vi "Default Section.vi"(8 "error in (no error)":errorcluster, 11 "Node Ptr":T1 format="%.0x") -> (0 "error out":errorcluster)   [LabVIEW 2019, in "Diagnostics Addon System Explorer.lvlib"]
uses:
  Diagnostics Addon System Explorer.lvlib
  <vilib>/NI VeriStand/Custom Device API/Custom Device Item Ref.ctl
  Addon Shared/SubVIs/Constants.vi
  <vilib>/NI VeriStand/Custom Device Tools/Custom Device Utility Library/NI VeriStand - Search for Item by GUID.vi
  <vilib>/NI VeriStand/Custom Device API/Custom Device API.lvlib
  <vilib>/NI VeriStand/Custom Device Tools/Custom Device Utility Library/Custom Device Utility Library.lvlib
  Addon Shared/Diagnostics Addon Shared.lvlib
panel:
  in  "SHDocVw.IWebBrowser":refnum<k7>(container)
  in  "Settings 6":i64 format="%.0x"
  in  "Settings 5":i64 format="%.0x"
  in  "Settings 4":i64 format="%.0x"
  in  "Settings 3":i64 format="%.0x"
  in  "Settings 2":i64 format="%.0x"
  in  "Settings 1":i64 format="%.0x"
  in  "Header 2":cluster{"Section Name":string}={"Section Name"="Section Default Values"}
  in  "Header":cluster{"Section Name":string}={"Section Name"="Section Item Settings"}
  in  "Description":string
  out "Name":string
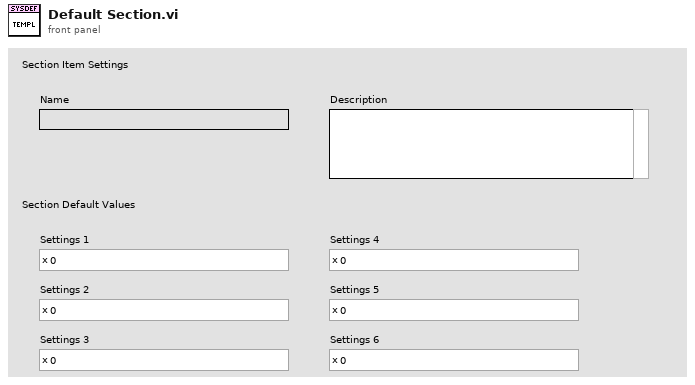
[diagram p1: front panel]
types:
  T1 = typedef "Custom Device API.lvlib/Custom Device Item Ref.ctl" = u64
  T2 = typedef "Custom Device API.lvlib/Custom Device Item Info.ctl" = cluster{"Name":string, "Is Channel":bool, "GUID":string, "Is Waveform":bool}
  T3 = typedef "Custom Device API.lvlib/Custom Device Channel.ctl" = cluster{"Type":T4, "Units":string, "Default Value":dbl, "Faultable":bool, "Scalable":bool}
  T4 = typedef "Custom Device API.lvlib/Custom Device Channel Type.ctl" = enum16{"Input", "Output"}
  T5 = typedef "Custom Device API.lvlib/Custom Device Commands.ctl" = enum16{"Default", "Item renamed", "Shutdown", "Dynamic button pressed"}
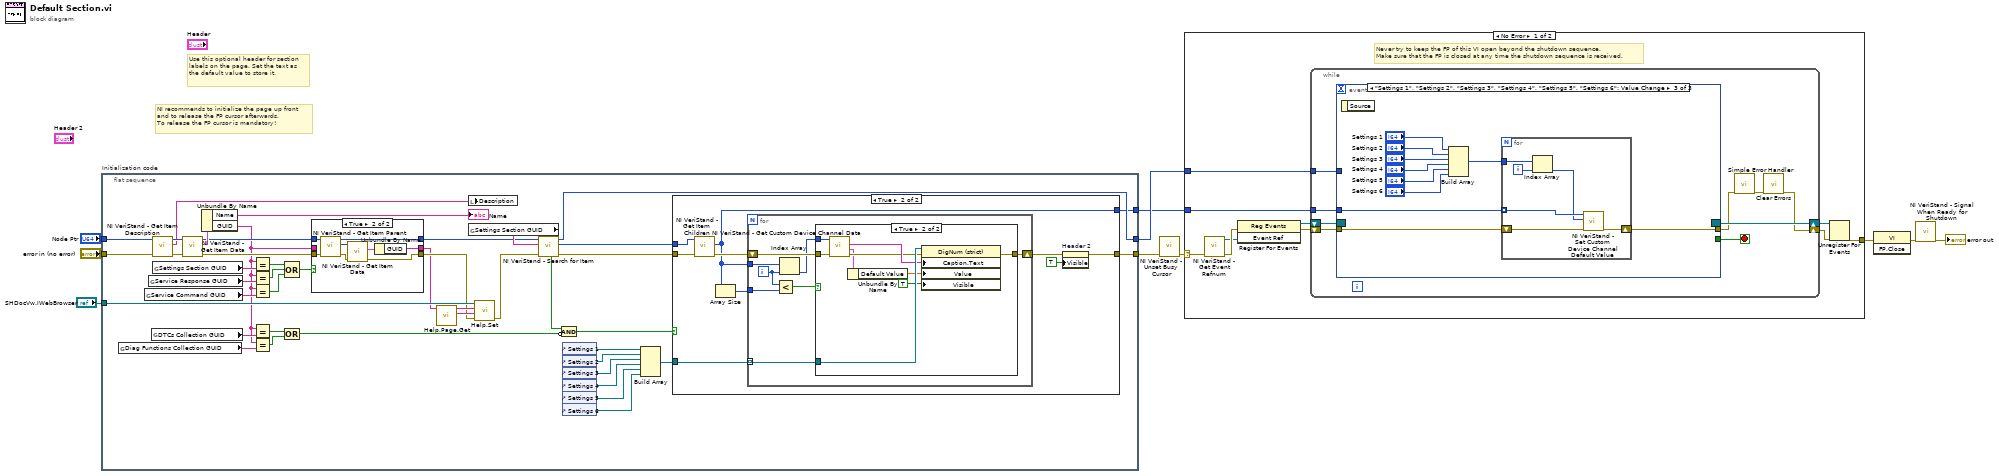
[diagram p0: block diagram]
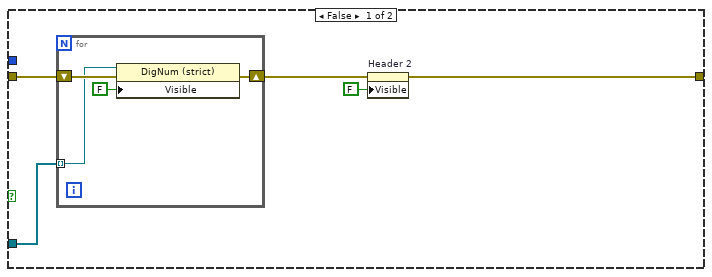
[diagram p3: hidden frame]
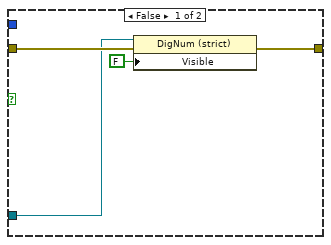
[diagram p4: hidden frame]
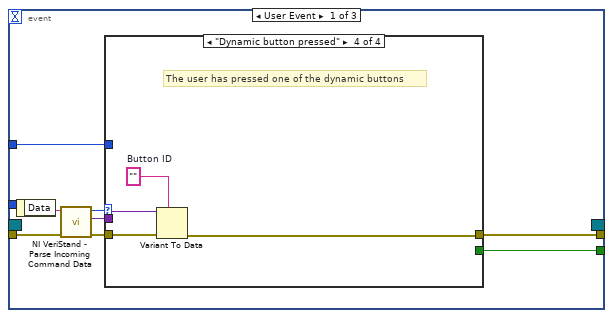
[diagram p5: hidden frame]
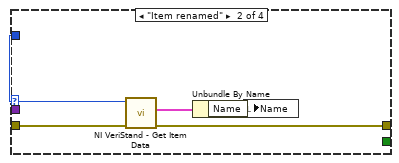
[diagram p7: hidden frame]
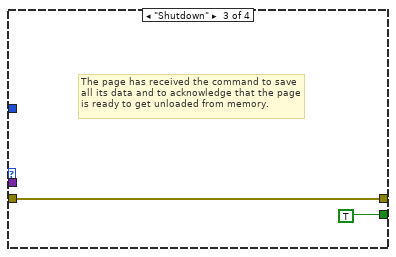
[diagram p8: hidden frame]
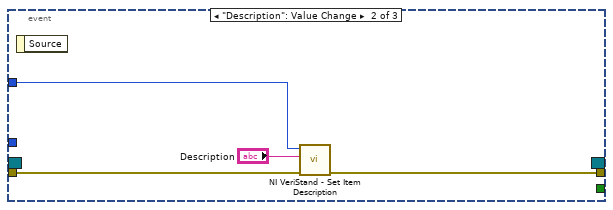
[diagram p9: hidden frame]
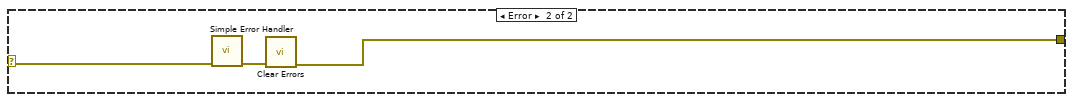
[diagram p10: hidden frame]
diagram:
  # "Use this optional header for section labels on the page. Set the text as the default value to store it."
  # "NI recommends to initialize the page up front\nand to release the FP cursor afterwards.\nTo release the FP cursor is mandatory!"
  n1 = flat-sequence "Initialization code" {
    tunnel: "error in (no error)" -> [w53]
    tunnel: "Node Ptr" -> [w52]
    tunnel: [w38] -> w6
    tunnel: [w37] -> w3
    tunnel: [w35] -> w2
    tunnel: "SHDocVw.IWebBrowser" -> [w33]
    frame #0 {
      n2 = global read "Constants.vi" "Diag Functions Collection GUID"() -> (w15:string)
      n3 = global read "Constants.vi" "Service Command GUID"() -> (w24:string)
      n4 = global read "Constants.vi" "Service Response GUID"() -> (w25:string)
      n5 = global read "Constants.vi" "DTCs Collection GUID"() -> (w16:string)
      n6 = call <vilib>:"NI VeriStand - Get Item Description.vi"("error in (no error)"=w53, "Item Ref in"=w52) -> ("error out"=w50:errorcluster, "Description"=w51:string, "Item Ref out"=w54:T1)  [unwired: 7 out]
      n7 = global read "Constants.vi" "Settings Section GUID"() -> (w23:string)
      n8 = call <vilib>:"NI VeriStand - Get Item Data.vi"("error in (no error)"=w50, "Item Ref in"=w54) -> ("error out"=w30:errorcluster, "Item Info"=w49:T2, "Item Ref out"=w29:T1)  [unwired: 7 out]
      n9 = Unbundle By Name(w49) -> ("Name"=→"Name":string, "GUID"=w14:string)
      n10 = Equal?(x=w14, y=w23) -> (x = y?=w20:bool)
      n11 = Equal?(x=w14, y=w25) -> (x = y?=w22:bool)
      n12 = Equal?(x=w14, y=w24) -> (x = y?=w21:bool)
      n13 = Equal?(x=w14, y=w16) -> (x = y?=w18:bool)
      n14 = Equal?(x=w14, y=w15) -> (x = y?=w17:bool)
      n15 = Compound Arithmetic op=OR(w20, w22, w21) -> (w19:bool)
      n16 = Compound Arithmetic op=OR(w18, w17) -> (w13:bool)
      n17 = case shown="True" w19 {
        tunnel: w30 -> [w57 w65]
        tunnel: w29 -> [w56 w64]
        tunnel: [w56 w63] -> w28
        tunnel: [w57 w59] -> w27
        tunnel: [w55 w58] -> w26
        tunnel: w14 -> [w55 _]
        frame False {
        }
        frame True {
          n18 = call <vilib>:"NI VeriStand - Get Item Parent.vi"("error in (no error)"=w65, "Item Ref in"=w64) -> ("error out"=w61:errorcluster, "Parent Ref"=w62:T1, "Item Ref out"=w63:T1)  [unwired: 6 in, 1 out]
          n19 = call <vilib>:"NI VeriStand - Get Item Data.vi"("error in (no error)"=w61, "Item Ref in"=w62) -> ("error out"=w59:errorcluster, "Item Info"=w60:T2)  [unwired: 8 out]
          n20 = Unbundle By Name(w60) -> ("GUID"=w58:string)
        }
      }
      n21 = call "Help.Page.Get.vi"("GUID"=w26) -> ("HTML File"=w34:string, "Main CHM File"=w31:string)  [unwired: 9 in]
      n22 = local write "Description"(w51) -> ()
      n23 = global read "Constants.vi" "Settings Section GUID"() -> (w47:string)
      n24 = call "Help.Set.vi"("error in (no error)"=w27, "HTML File"=w34, "Main CHM File"=w31, "SHDocVw.IWebBrowser2"=w33) -> ("error out"=w32:errorcluster)  [unwired: 7 in]
      n25 = call-poly <vilib>:"NI VeriStand - Search for Item.vi"("error in"=w32, "Item GUID"=w47, "Section Ref in"=w28) -> ("error out"=w39:errorcluster, "Item Ref"=w36:T1, "Section Ref out"=w37:T1, "Found"=w12:bool)  [unwired: 5 in]
      n26 = Compound Arithmetic op=AND(w12, invert w13) -> (w11:bool)
      n27 = control-ref of="Settings 1"() -> (w46:refnum<vi>)
      n28 = control-ref of="Settings 2"() -> (w45:refnum<vi>)
      n29 = control-ref of="Settings 3"() -> (w44:refnum<vi>)
      n30 = control-ref of="Settings 4"() -> (w43:refnum<vi>)
      n31 = control-ref of="Settings 5"() -> (w42:refnum<vi>)
      n32 = control-ref of="Settings 6"() -> (w41:refnum<vi>)
      n33 = Build Array(w46, w45, w44, w43, w42, w41) -> (w40:refnum<vi>[])
      n34 = case shown="True" w11 {
        tunnel: w40 -> [w70 w83]
        tunnel: w39 -> [w69 w82]
        tunnel: [w66 w75] -> w38
        tunnel: w36 -> [_ w80]
        tunnel: [_ w78] -> w35
        frame False {
          n35 = for {
            tunnel: w70 -> [w73] mode=indexing
            shift-right: [w71] -> w67
            shift-left: w69 -> [w74]
            n36 = property class="DigNum (strict)"(reference=w73, error in=w74, "Visible"=FALSE) -> (error out=w71:errorcluster)  [unwired: 1 out]
          }
          n37 = property on="Header 2" class="Clust (strict)"(error in=w67, "Visible"=FALSE) -> (error out=w66:errorcluster)  [unwired: 1 in, 1 out]
        }
        frame True {
          n38 = call <vilib>:"NI VeriStand - Get Item Children.vi"("error in (no error)"=w82, "Item Ref in"=w80) -> ("error out"=w81:errorcluster, "Child Refs"=w78:T1[])  [unwired: 6 in, 2 out]
          n39 = Array Size(array=w78) -> (size(s)=w79:i32)
          n40 = for {
            tunnel: w83 -> [w91] mode=indexing
            shift-right: [w90] -> w76
            shift-left: w81 -> [w88]
            tunnel: w78 -> [w89]
            tunnel: w79 -> [w85]
            i -> [w86]
            n41 = Less?(x=w86, y=w85) -> (x < y?=w84:bool)
            n42 = Index Array(array=w89, index=w86) -> (element=w87:T1)
            n43 = case shown="True" w84 {
              tunnel: w91 -> [w92 w104]
              tunnel: [w93 w103] -> w90
              tunnel: w88 -> [w94 w101]
              tunnel: w87 -> [_ w100]
              frame False {
                n44 = property class="DigNum (strict)"(reference=w92, error in=w94, "Visible"=FALSE) -> (error out=w93:errorcluster)  [unwired: 1 out]
              }
              frame True {
                n45 = call <vilib>:"NI VeriStand - Get Custom Device Channel Data.vi"("error in (no error)"=w101, "Channel Ref in"=w100) -> ("error out"=w98:errorcluster, "Channel"=w97:T3, "Channel Name"=w99:string)  [unwired: 4 in, 3 out]
                n46 = Unbundle By Name(w97) -> ("Default Value"=w96:dbl)
                n47 = property class="DigNum (strict)"(reference=w104, error in=w98, "Caption.Text"=w99, "Value"=w96, "Visible"=TRUE) -> (error out=w103:errorcluster)  [unwired: 1 out]
              }
            }
          }
          n48 = property on="Header 2" class="Clust (strict)"(error in=w76, "Visible"=TRUE) -> (error out=w75:errorcluster)  [unwired: 1 in, 1 out]
        }
      }
    }
  }
  n49 = call <vilib>:"NI VeriStand - Unset Busy Cursor.vi"("error in (no error)"=w6) -> ("error out"=w5:errorcluster)  [unwired: 10 out]
  n50 = case shown="No Error" w5 {
    selector: w5 -> [w106 w166]
    tunnel: [w111 w164] -> w10
    tunnel: w3 -> [w107 _]
    tunnel: w2 -> [w105 _]
    frame No Error {
      # "Never try to keep the FP of this VI open beyond the shutdown sequence.\nMake sure that the FP is closed at any time the shutdown sequence is received."
      n51 = call <vilib>:"NI VeriStand - Get Event Refnum.vi"("error in (no error)"=w106) -> ("error out"=w114:errorcluster, "Event Ref"=w110:refnum<user-event>)  [unwired: 9 out]
      n52 = register-events(error in=w114, w110) -> (reference out=w108:refnum<event-registration>, error out=w109:errorcluster)  [unwired: 1 in]
      n53 = while {
        tunnel: w107 -> [w119]
        shift-right: [w116] -> w112
        shift-left: w109 -> [w122]
        shift-right: [w123] -> w113
        shift-left: w108 -> [w121]
        tunnel: w105 -> [w115]
        stop <- w120 stop-if-true
        n54 = event shown="[2] \"Settings 1\", \"Settings 2\", \"Settings 3\", \"Settings 4\", \"Settings 5\", \"Settings 6\": Value Change" {
          selector: w121 -> [_ _ _]
          dyn-events: [_ _ _] -> w123
          timeout: _ -> [_ _ _]
          tunnel: w122 -> [w131 w146 w157]
          tunnel: [w127 _ _] -> w120
          tunnel: [w126 w145 w155] -> w118
          tunnel: w119 -> [w125 w147 _]
          tunnel: w115 -> [_ _ w156]
          event User Event {
            n55 = event-data() -> ("Data"=w130:string)  [unwired: 1 out]
            n56 = call <vilib>:"NI VeriStand - Parse Incoming Command Data.vi"("error in (no error)"=w131, "Incoming data"=w130) -> ("error out"=w129:errorcluster, "Outgoing data"=w124:variant, "Action"=w128:T5)  [unwired: 7 out]
            n57 = case shown="\"Dynamic button pressed\"" w128 {
              tunnel: w129 -> [w132 w137 w138 w143]
              tunnel: [_ _ TRUE _] -> w127
              tunnel: [w132 w134 w138 w140] -> w126
              tunnel: w125 -> [_ w136 _ _]
              tunnel: w124 -> [_ _ _ w142]
              frame "Default", Default {
              }
              frame "Item renamed" {
                n58 = call <vilib>:"NI VeriStand - Get Item Data.vi"("error in (no error)"=w137, "Item Ref in"=w136) -> ("error out"=w134:errorcluster, "Item Info"=w135:T2)  [unwired: 8 out]
                n59 = Unbundle By Name(w135) -> ("Name"=w133:string)
                n60 = local write "Name"(w133) -> ()
              }
              frame "Shutdown" {
                # "The page has received the command to save all its data and to acknowledge that the page is ready to get unloaded from memory."
              }
              frame "Dynamic button pressed" {
                w141 = ""  # Button ID
                # "The user has pressed one of the dynamic buttons"
                n61 = Variant To Data(error in=w143, type=w141, Variant=w142) -> (error out=w140:errorcluster)  [unwired: 1 out]
              }
            }
          }
          event "Description": Value Change {
            n62 = event-data() -> ()  [unwired: 2 out]
            n63 = call <vilib>:"NI VeriStand - Set Item Description.vi"("error in (no error)"=w146, "Description"="Description", "Item Ref in"=w147) -> ("error out"=w145:errorcluster)  [unwired: 8 out]
          }
          event "Settings 1", "Settings 2", "Settings 3", "Settings 4", "Settings 5", "Settings 6": Value Change {
            n64 = event-data() -> ()  [unwired: 2 out]
            n65 = Build Array("Settings 1", "Settings 2", "Settings 3", "Settings 4", "Settings 5", "Settings 6") -> (w148:i64[])
            n66 = for {
              tunnel: w156 -> [w162] mode=indexing
              shift-right: [w161] -> w155
              shift-left: w157 -> [w163]
              tunnel: w148 -> [w160]
              i -> [w158]
              n67 = Index Array(array=w160, index=w158) -> (element=w159:i64)
              n68 = call <vilib>:"NI VeriStand - Set Custom Device Channel Default Value.vi"("error in (no error)"=w163, "Default Value"=w159, "Channel Ref in"=w162) -> ("error out"=w161:errorcluster)  [unwired: 7 in, 1 out]
            }
          }
        }
        n69 = call <vilib>:"Simple Error Handler.vi"("error in (no error)"=w118) -> ("error out"=w117:errorcluster)  [unwired: 1 in, 7 out]
        n70 = call <vilib>:"Clear Errors.vi"("error in (no error)"=w117) -> ("error out"=w116:errorcluster)  [unwired: 1 in, 5 out]
      }
      n71 = Unregister For Events(event registration refnum=w113, error in=w112) -> (error out=w111:errorcluster)
    }
    frame Error {
      n72 = call <vilib>:"Simple Error Handler.vi"("error in (no error)"=w166) -> ("error out"=w165:errorcluster)  [unwired: 1 in, 7 out]
      n73 = call <vilib>:"Clear Errors.vi"("error in (no error)"=w165) -> ("error out"=w164:errorcluster)  [unwired: 1 in, 5 out]
    }
  }
  n74 = invoke class="VI" method="FP.Close"(error in=w10) -> (error out=w9:errorcluster)  [unwired: 2 in, 2 out]
  n75 = call <vilib>:"NI VeriStand - Signal When Ready for Shutdown.vi"("error in (no error)"=w9) -> ("error out"=→"error out":errorcluster)  [unwired: 10 out]
